vi "Initialize.vi"(8 "error in (no error)":errorcluster, 9 "Components":refnum<class "Component.lvclass">[](array[class]), 10 "framework configuration":T1={"plugins"=[{"name"="Plugin", "components"=[], "cycle timing"={"priority"=10000, "decimation"=1, "offset"=0}, "threads"=[{"core"={"processor"=-2, "priority offset"=0}, "component settings"=[], "transfer groups"=[]}, {"core"={"processor"=-2, "priority offset"=0}, "component settings"=[], "transfer groups"=[]}, {"core"={"processor"=-2, "priority offset"=0}, "component settings"=[], "transfer groups"=[]}, {"core"={"processor"=-2, "priority offset"=0}, "component settings"=[], "transfer groups"=[]}], "transfer groups"=[], "settings"=[]}]}, 11 "Framework Configuration in":refnum<class "Framework Configuration.lvclass">) -> (0 "error out":errorcluster, 3 "Framework Configuration out":refnum<class "Framework Configuration.lvclass">)   [LabVIEW 2017, in "DSF Core.lvlib" / "Framework Configuration.lvclass"]
uses:
  Framework Configuration.lvclass
  DSF Core.lvlib
  Base/Plugin/Plugin Configuration.lvclass
  Core/Framework/Core Framework Configuration.lvclass
  Typedefs/DSF Engine Framework Configuration.ctl
  Component/Component.lvclass
  Typedefs/DSF Timing Info.ctl
  Typedefs/DSF Settings Info.ctl
  Typedefs/DSF Engine Plugin Thread Configuration.ctl
  Typedefs/DSF Direction.ctl
  Typedefs/DSF Data Type.ctl
  Typedefs/DSF Engine Channel Configuration.ctl
  Typedefs/DSF Engine Transfer Configuration.ctl
  Typedefs/DSF Timeout Behavior.ctl
  Typedefs/DSF Engine Transfer Group Configuration.ctl
  Typedefs/DSF Engine Plugin Configuration.ctl
  Typedefs/DSF Version Info.ctl
  Typedefs/DSF Core Channel Configuration.ctl
  Typedefs/DSF Core Transfer Configuration.ctl
  Typedefs/DSF Core Group Configuration.ctl
  Typedefs/DSF Core Thread Configuration.ctl
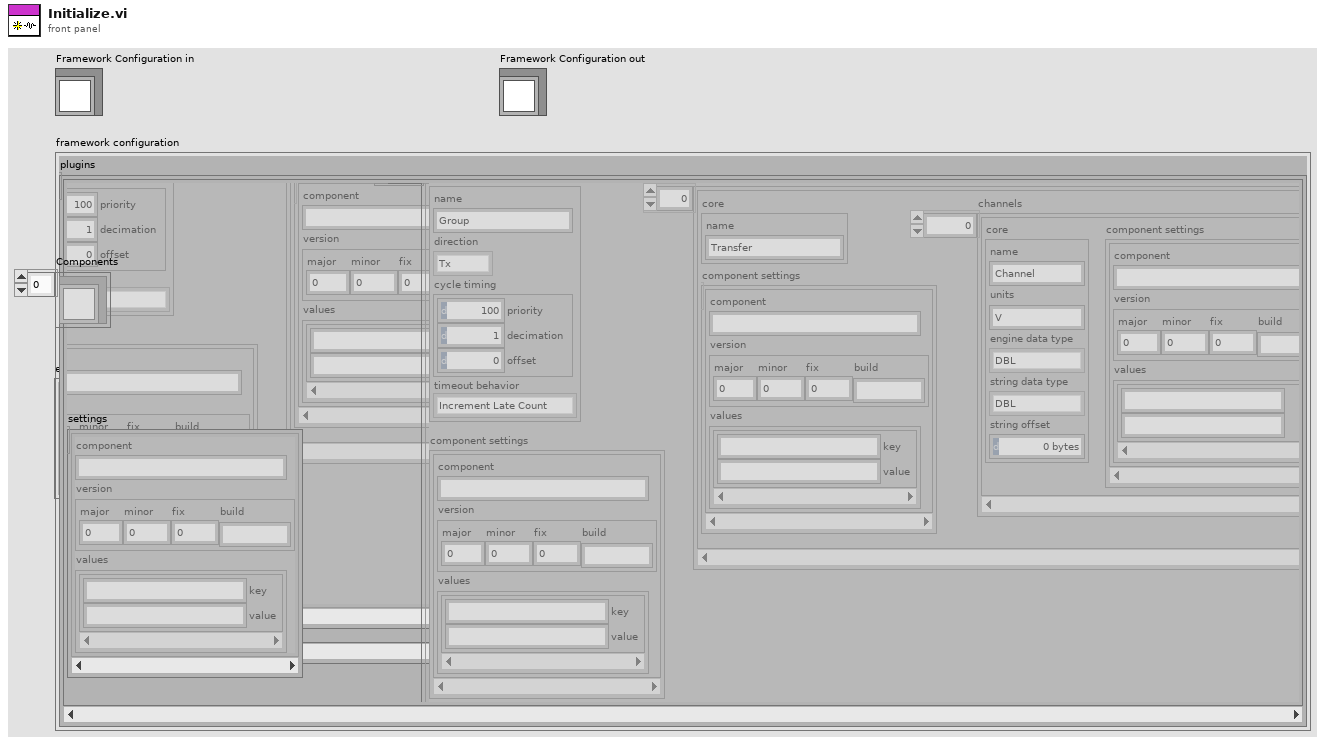
[diagram p1: front panel]
types:
  T1 = typedef "DSF Core.lvlib/DSF Engine Framework Configuration.ctl" = cluster{"plugins":T2[]}
  T2 = typedef "DSF Core.lvlib/DSF Engine Plugin Configuration.ctl" = cluster{"name":string, "components":string[], "cycle timing":T3, "threads":T4[], "transfer groups":T8[], "settings":T6}
  T3 = typedef "DSF Core.lvlib/DSF Timing Info.ctl" = cluster{"priority":u64, "decimation":u64, "offset":u64}
  T4 = typedef "DSF Core.lvlib/DSF Engine Plugin Thread Configuration.ctl" = cluster{"core":T5, "component settings":T6, "transfer groups":T8[]}
  T5 = typedef "DSF Core.lvlib/DSF Core Thread Configuration.ctl" = cluster{"processor":i32, "priority offset":i16}
  T6 = typedef "DSF Core.lvlib/DSF Settings Info.ctl" = cluster{"component":string, "version":T7, "values":cluster{"key":string, "value":string}[]}[]
  T7 = typedef "DSF Core.lvlib/DSF Version Info.ctl" = cluster{"major":u32, "minor":u32, "fix":u32, "build":string}
  T8 = typedef "DSF Core.lvlib/DSF Engine Transfer Group Configuration.ctl" = cluster{"core":T9, "component settings":T6, "transfers":T12[]}
  T9 = typedef "DSF Core.lvlib/DSF Core Group Configuration.ctl" = cluster{"name":string, "direction":T10, "cycle timing":T3, "timeout behavior":T11}
  T10 = typedef "DSF Core.lvlib/DSF Direction.ctl" = enum8{"Tx", "Rx"}
  T11 = typedef "DSF Core.lvlib/DSF Timeout Behavior.ctl" = enum8{"Increment Late Count", "Throw Error"}
  T12 = typedef "DSF Core.lvlib/DSF Engine Transfer Configuration.ctl" = cluster{"core":T13, "component settings":T6, "channels":T14[]}
  T13 = typedef "DSF Core.lvlib/DSF Core Transfer Configuration.ctl" = cluster{"name":string}
  T14 = typedef "DSF Core.lvlib/DSF Engine Channel Configuration.ctl" = cluster{"core":T15, "component settings":T6}
  T15 = typedef "DSF Core.lvlib/DSF Core Channel Configuration.ctl" = cluster{"name":string, "units":string, "engine data type":T16, "string data type":T16, "string offset":u64}
  T16 = typedef "DSF Core.lvlib/DSF Data Type.ctl" = enum8{"Bool", "SGL", "DBL", "I8", "I16", "I32", "I64", "U8", "U16", "U32", "U64"}
  T17 = typedef "DSF Core.lvlib/DSF Component Configuration.ctl" = cluster{"component":string, "data":string, "data version":T18}
  T18 = typedef "DSF Core.lvlib/DSF Version Info.ctl" = cluster{"major":i32, "minor":i32, "fix":i32, "build":string}
  T19 = typedef "DSF Core.lvlib/DSF Component Configuration.ctl" = cluster{"component":string, "data":string, "data version":T7}
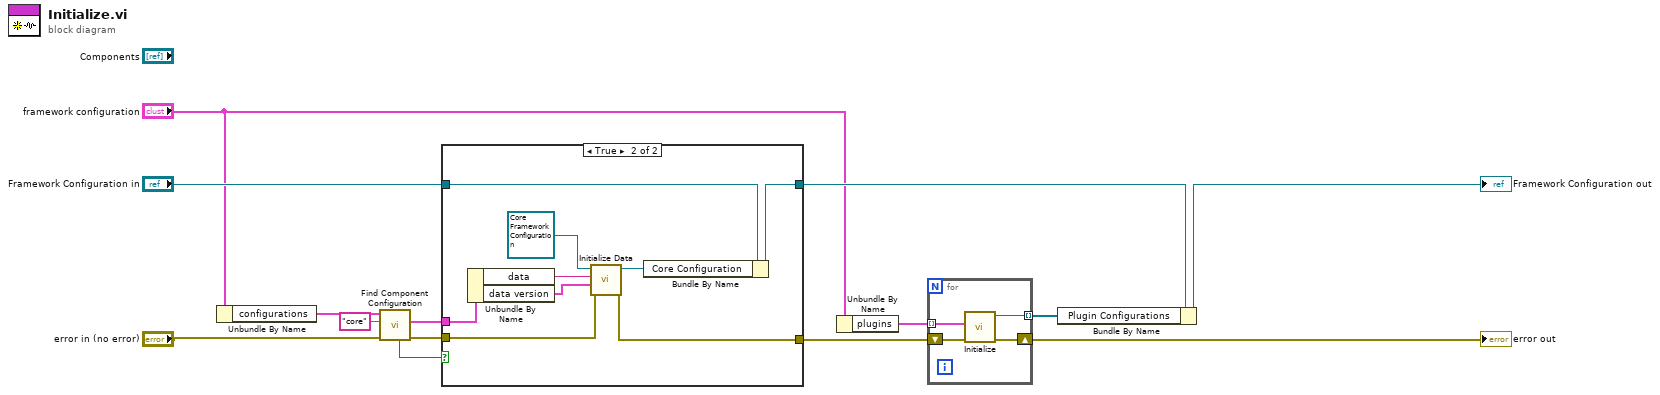
[diagram p0: block diagram]
diagram:
  n1 = Unbundle By Name("framework configuration") -> ("configurations"=w12:T17[])
  n2 = call "Find Component Configuration.vi"("error in (no error)"="error in (no error)", "component"="core", "configurations in"=w12) -> ("error out"=w10:errorcluster, "component configuration"=w8:T19, "found?"=w9:bool)  [unwired: 4 in, 2 out]
  n3 = case shown="True" w9 {
    tunnel: "Framework Configuration in" -> [w16 w18]
    tunnel: [w16 w19] -> w5
    tunnel: [w15 w20] -> w6
    tunnel: w10 -> [w15 w23]
    tunnel: w8 -> [_ w21]
    frame False {
    }
    frame True {
      n4 = Unbundle By Name(w21) -> ("data"=w24:string, "data version"=w25:T7)
      n5 = call-dynamic "Initialize Data.vi"("error in (no error)"=w23, "data version"=w25, "data"=w24, "Configuration in"=refnum<class "Core Framework Configuration.lvclass"> refnum ("Core Configuration")) -> ("error out"=w20:errorcluster, "Configuration out"=w17:refnum<class "Core Framework Configuration.lvclass">)  [unwired: 6 in]
      n6 = Bundle By Name(cluster=w18, "Core Configuration"=w17) -> (w19:refnum<class "Framework Configuration.lvclass">)
    }
  }
  n7 = Unbundle By Name("framework configuration") -> ("plugins"=w3:T2[])
  n8 = for {
    tunnel: [w28] -> w7 mode=indexing
    shift-right: [w27] -> w1
    shift-left: w6 -> [w29]
    tunnel: w3 -> [w26] mode=indexing
    n9 = call "Initialize.vi"("error in (no error)"=w29, "plugin configuration"=w26) -> ("error out"=w27:errorcluster, "Plugin Configuration out"=w28:refnum<class "Plugin Configuration.lvclass">)  [unwired: 8 in]
  }
  "error out" <- w1
  n10 = Bundle By Name(cluster=w5, "Plugin Configurations"=w7) -> (→"Framework Configuration out":refnum<class "Framework Configuration.lvclass">)
